vi "slider setter.vi"(6 "stepper motor state":T2, 7 "slider setter action":T3, 8 "state in":T1, 10 "value":dbl=1.0 format="%#_13g") -> (0 "state OUT":T1)   [LabVIEW 2018]
uses:
  slider setter action.ctl
  stepper motor state.ctl
  slider setter interal state.ctl
  2Dwindow.ctl
  stack action -- control.ctl
  slider action.ctl
  cursor action.ctl
  generate linear region.vi
  generate linear region --complex -- win cen.vi
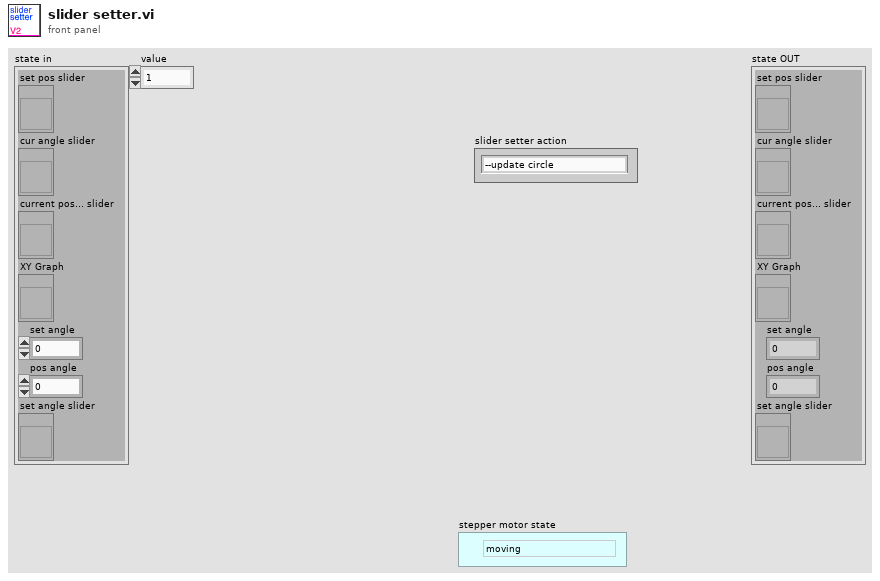
[diagram p1: front panel]
types:
  T1 = typedef "slider setter interal state.ctl" = cluster{"set pos slider":refnum<vi>, "cur angle slider":refnum<vi>, "current pos... slider":refnum<vi>, "XY Graph":refnum<vi>, "set angle":dbl, "pos angle":dbl, "set angle slider":refnum<vi>}
  T2 = typedef "stepper motor state.ctl" = enum16{"moving", "stopped"}
  T3 = typedef "slider setter action.ctl" = enum16{"--update circle", "set step slider moves", "cursor moves", "current pos changed", "init", "void", "--draw current lie", "--draw set line", "--move current step slider", "--move set step slider", "--draw limit lines", "check", "--move set angle slider", "--move current angle slider", "set angle slider moves", "--move cursor", "set set step", "set current step"}
  T4 = typedef "stack action -- control.ctl" = enum16{"push", "pop", "check", "init"}
  T5 = typedef "2Dwindow.ctl" = cluster{"window y":dbl, "center x":dbl, "center y":dbl, "window x":dbl}
  T6 = typedef "slider action.ctl" = enum16{"check", "copy range", "set from value", "set from ratio", "set from slider"}
  T7 = typedef "cursor action.ctl" = enum16{"range", "read", "write", "check", "zoom out", "smart zoom out", "zoom to aspect ratio 1", "zoom to win", "zoom out 20%", "zoom in 20%", "-empty", "smart zoom out&aspect", "move range left 20%", "move range right 20%", "move range up 20%", "move range down 20%", "zoom to X win", "zoom to Y win", "zoom out X", "zoom out Y", "zoom in X", "zoom in Y", "check plot scale"}
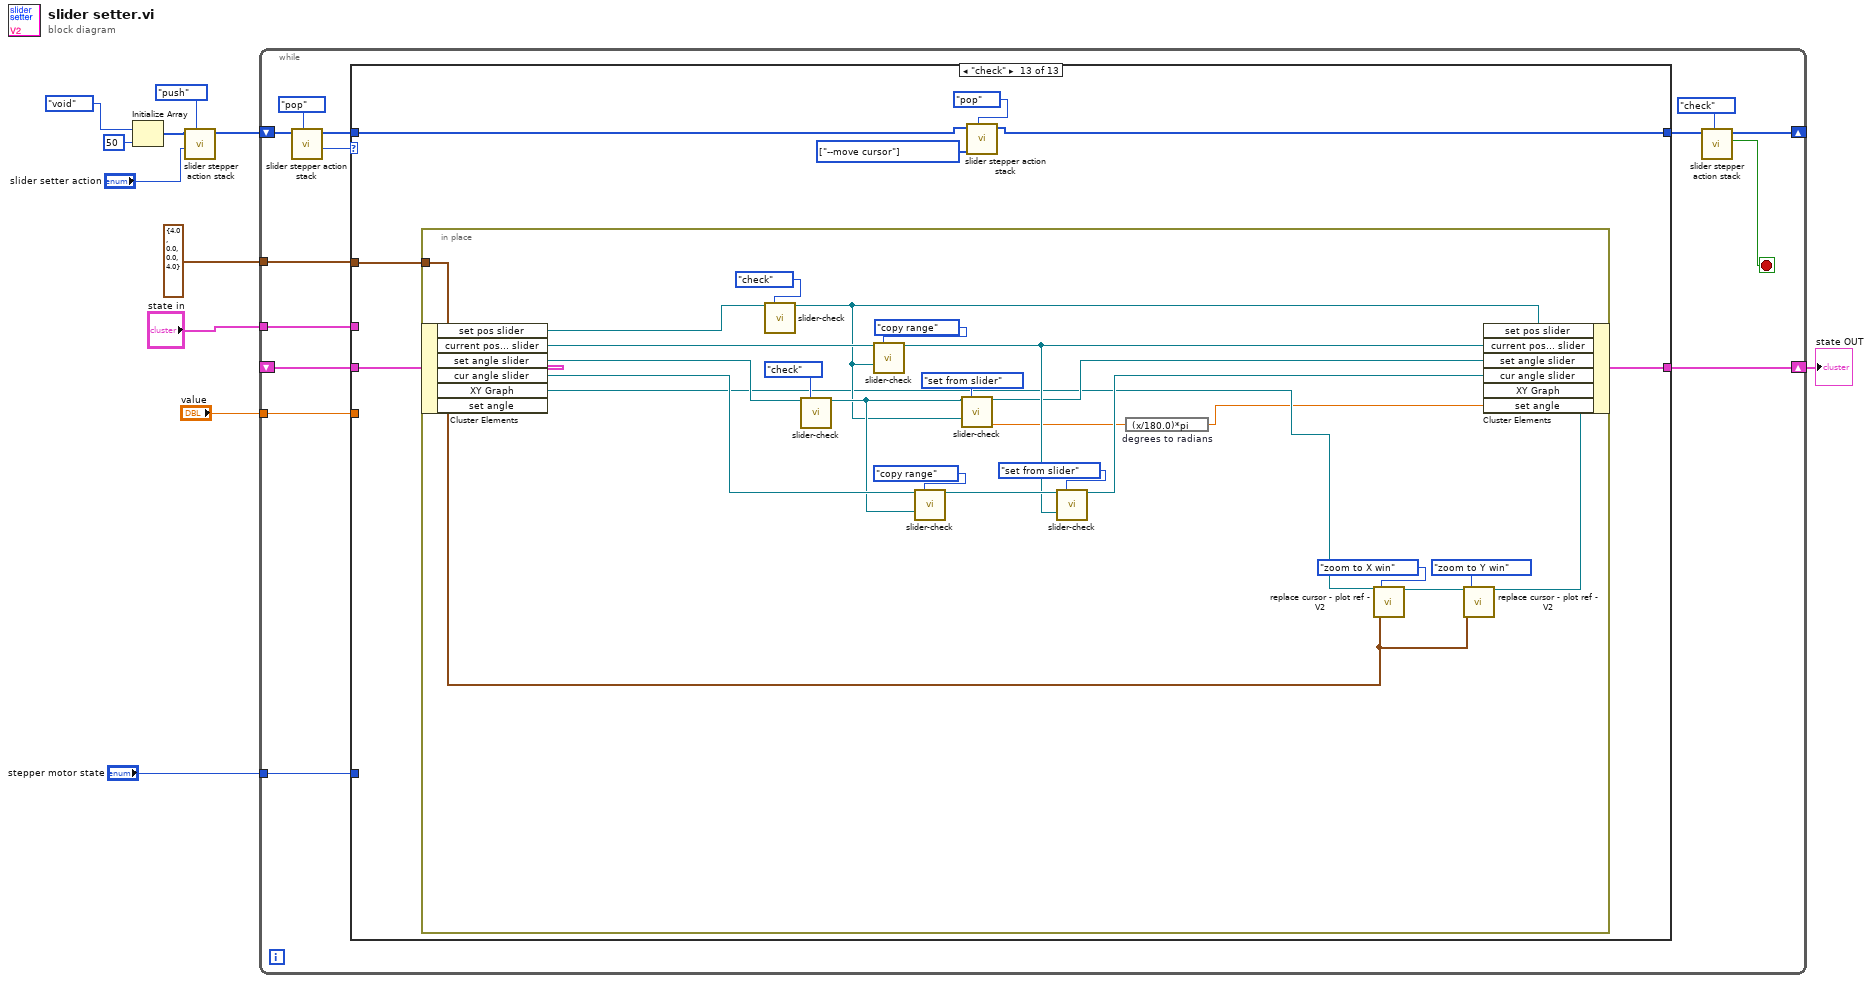
[diagram p0: block diagram]
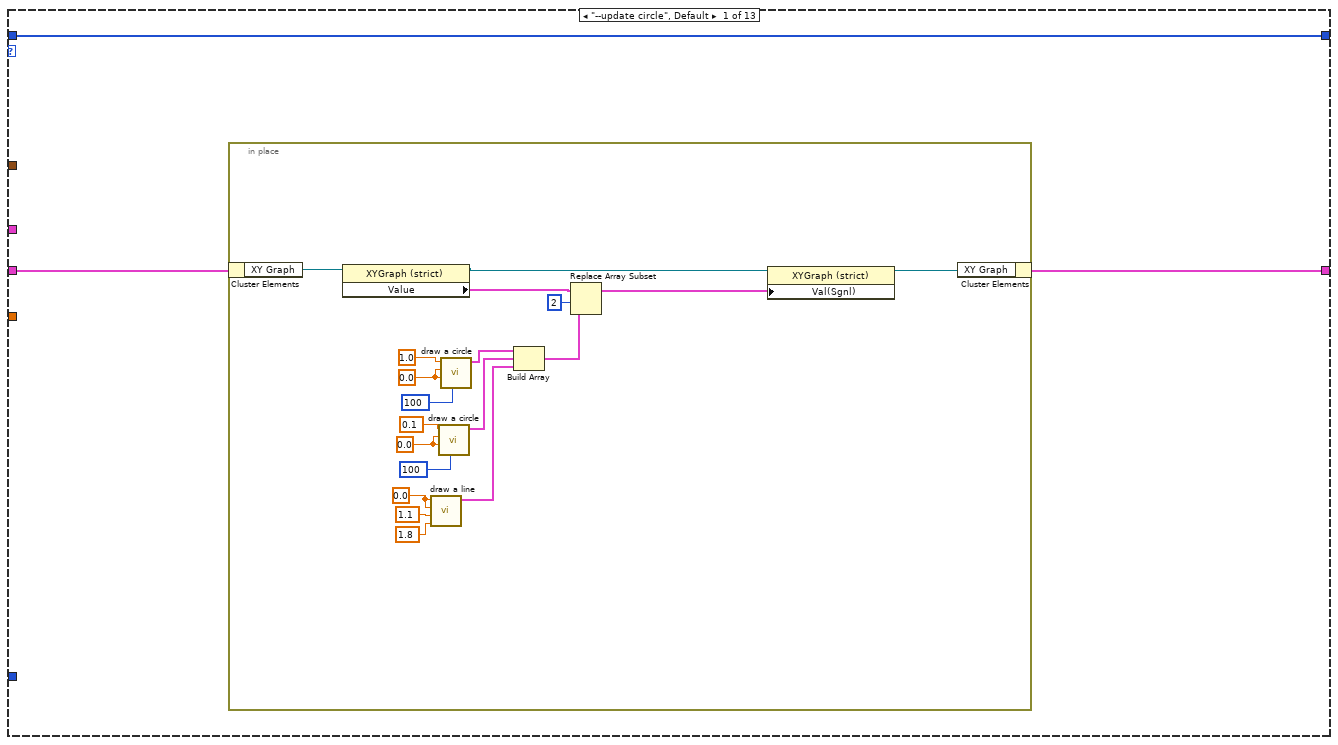
[diagram p2: hidden frame]
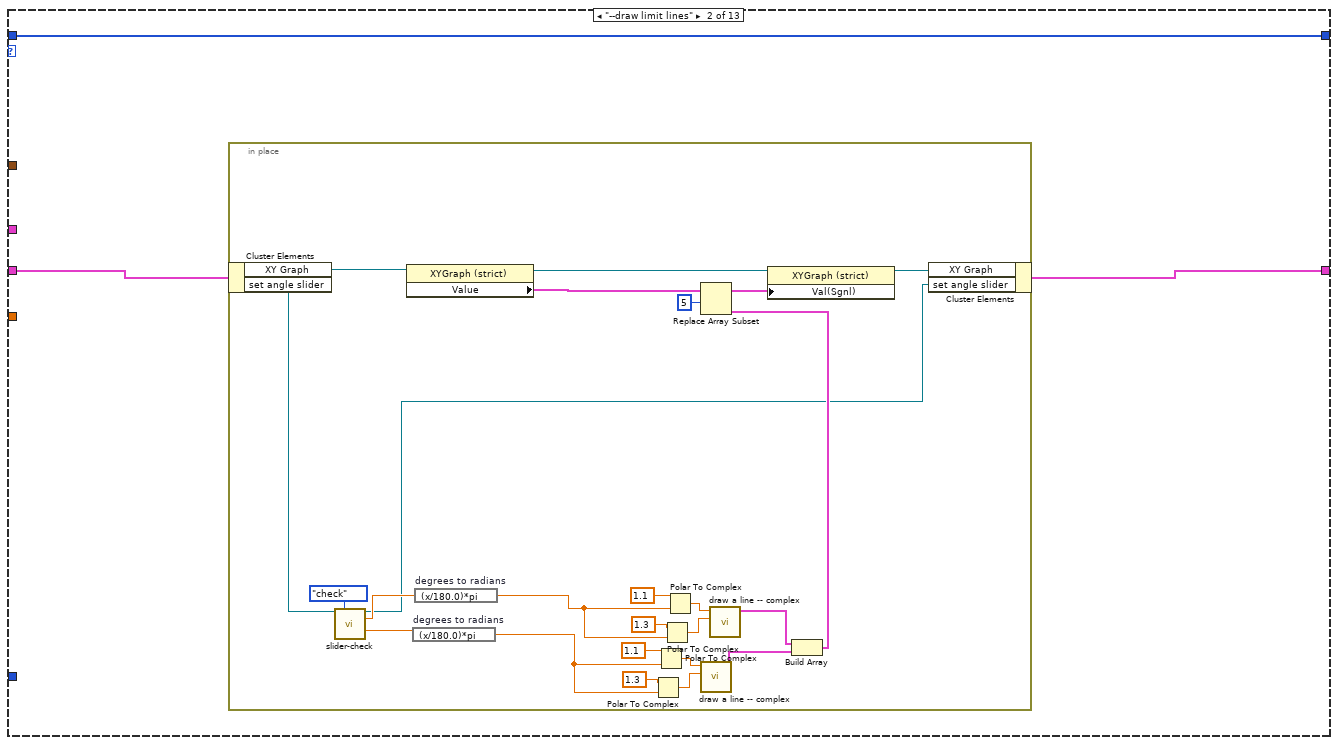
[diagram p3: hidden frame]
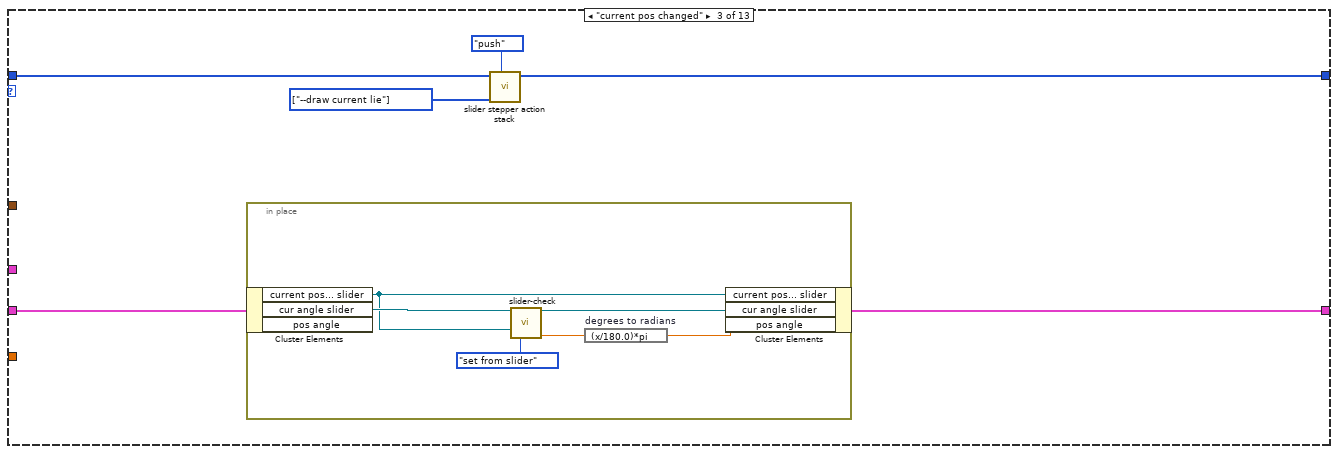
[diagram p4: hidden frame]
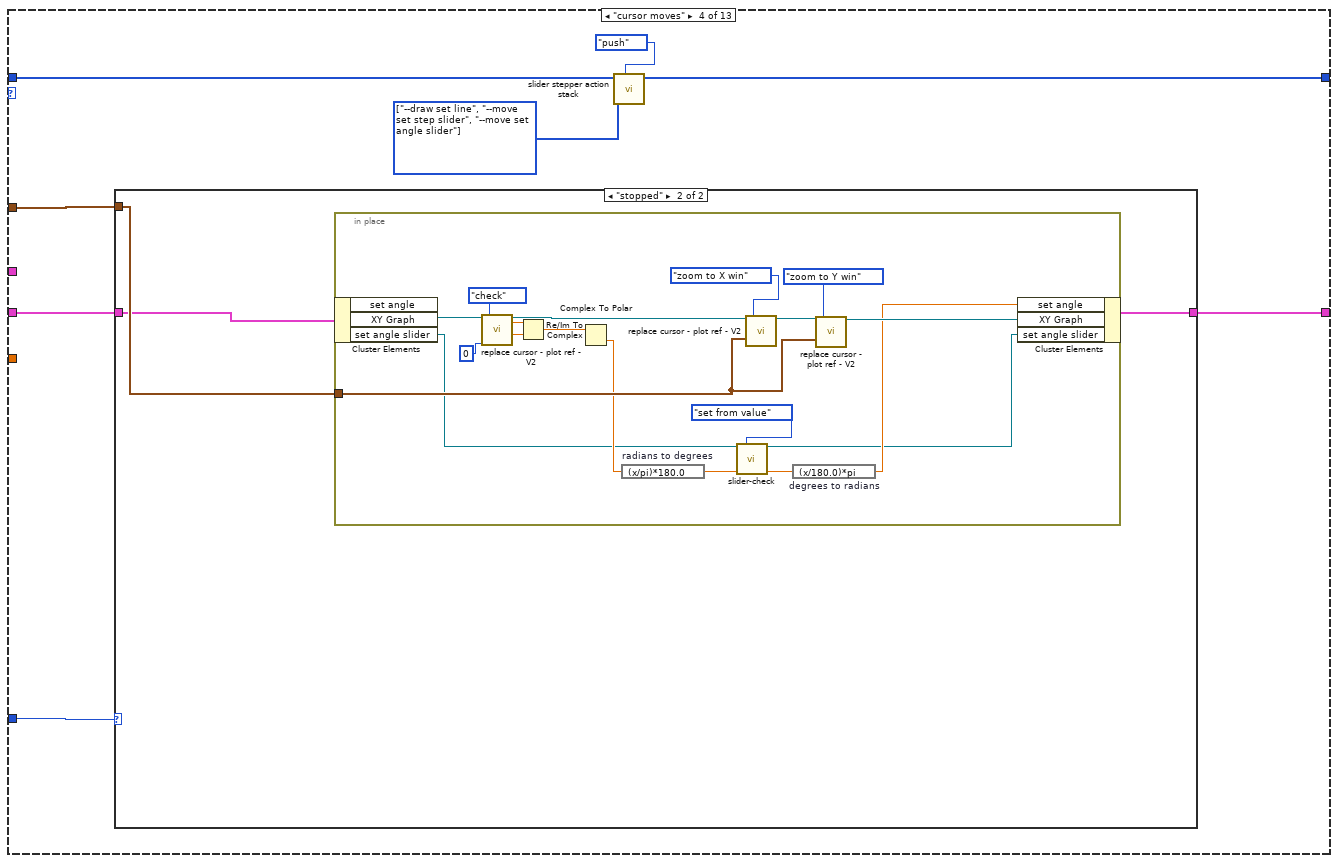
[diagram p5: hidden frame]
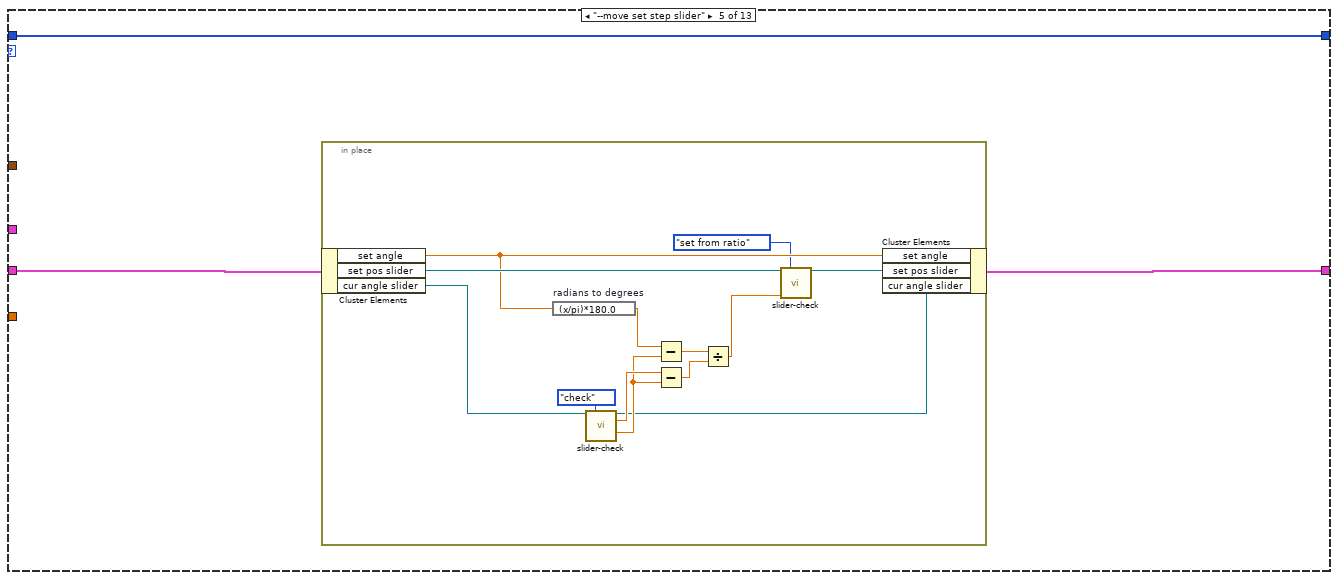
[diagram p7: hidden frame]
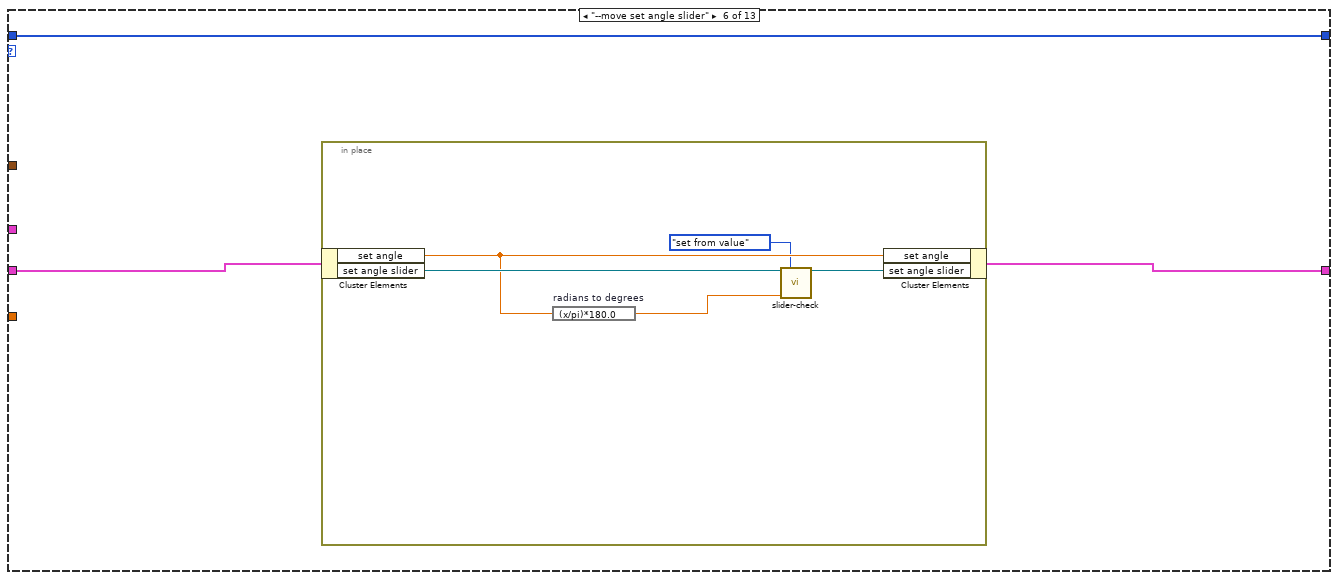
[diagram p8: hidden frame]
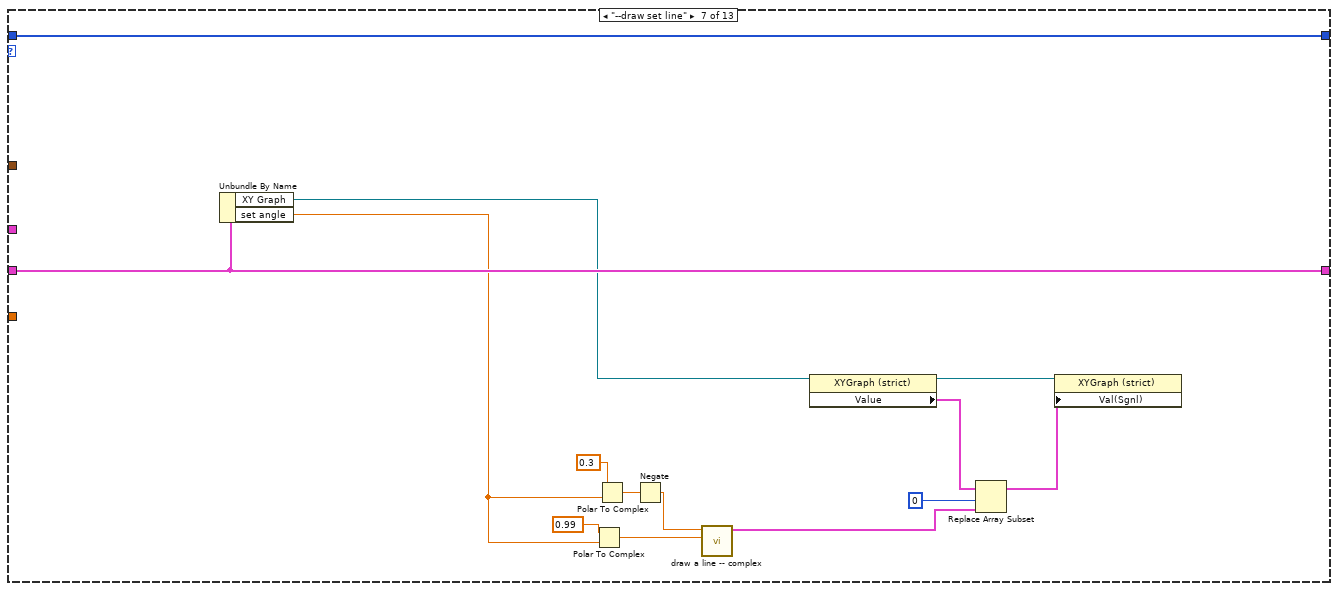
[diagram p9: hidden frame]
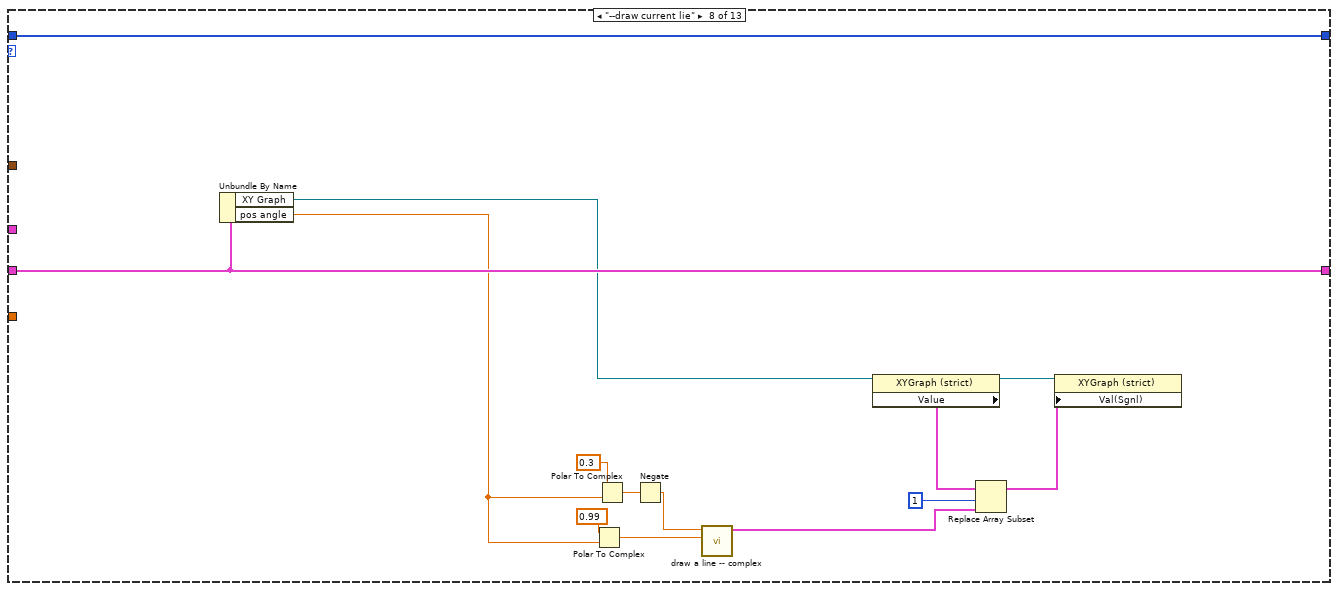
[diagram p10: hidden frame]
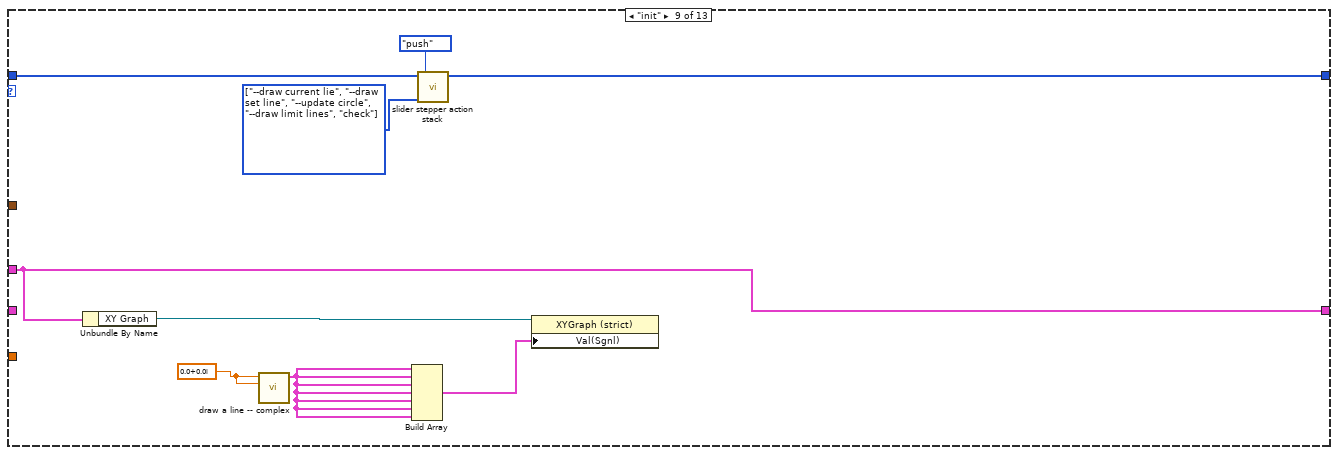
[diagram p11: hidden frame]
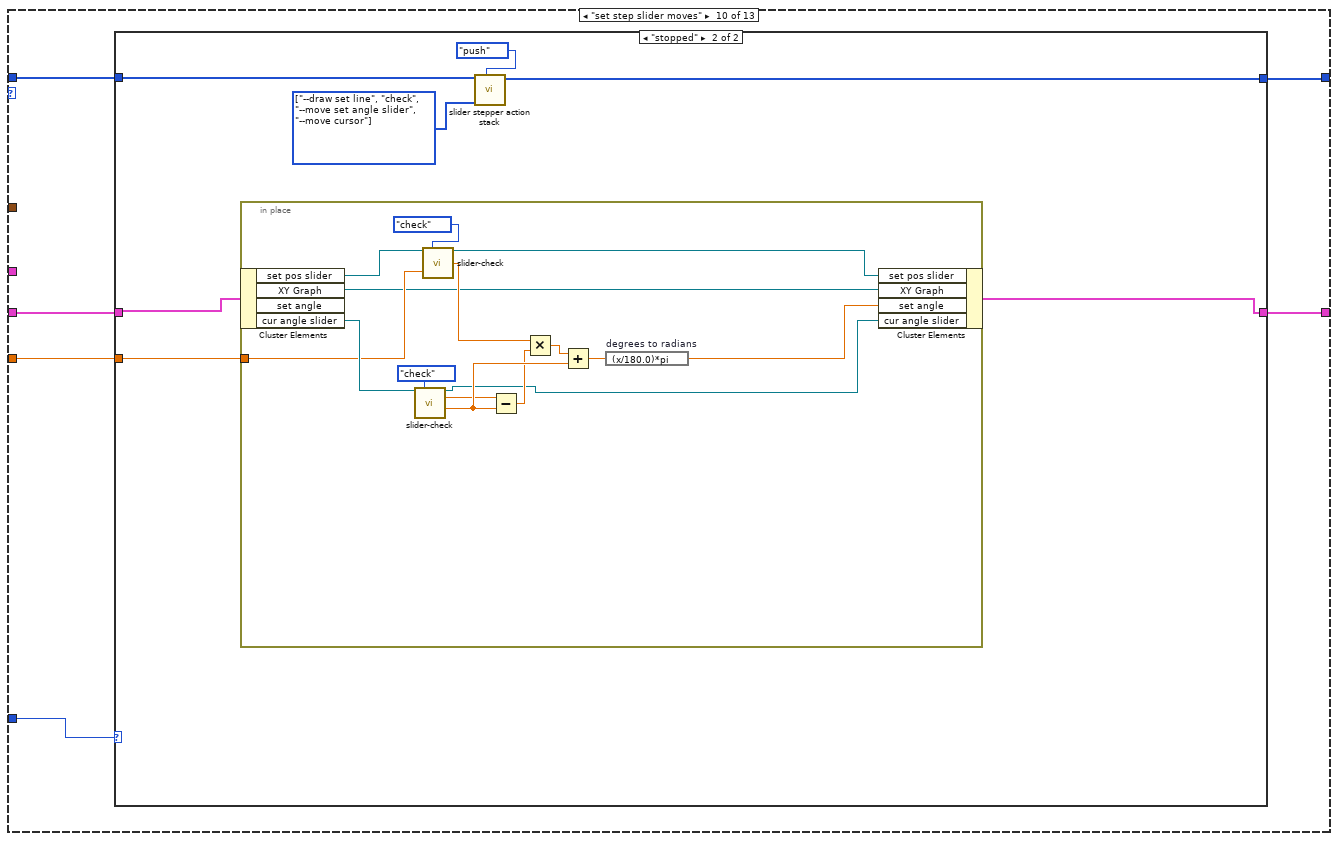
[diagram p12: hidden frame]
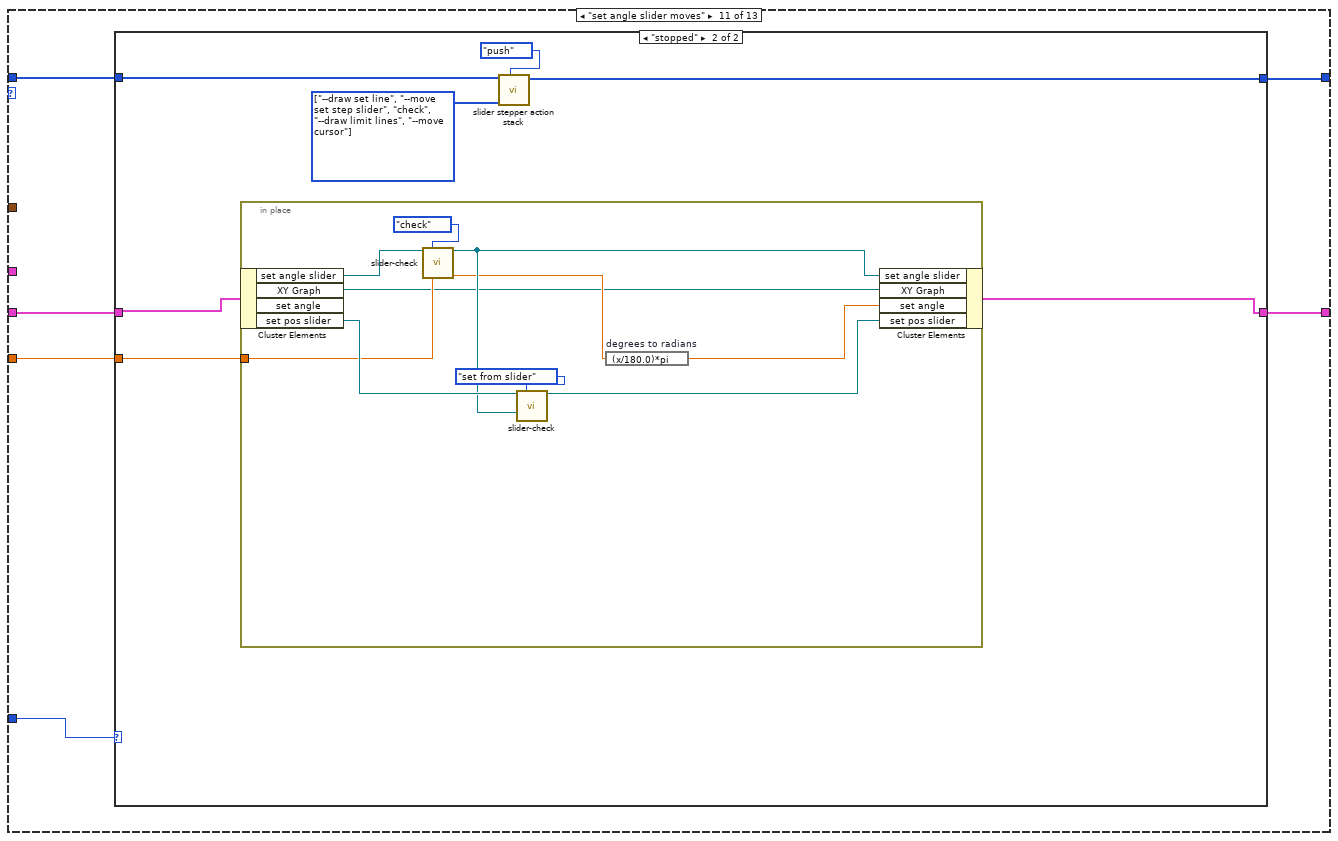
[diagram p14: hidden frame]
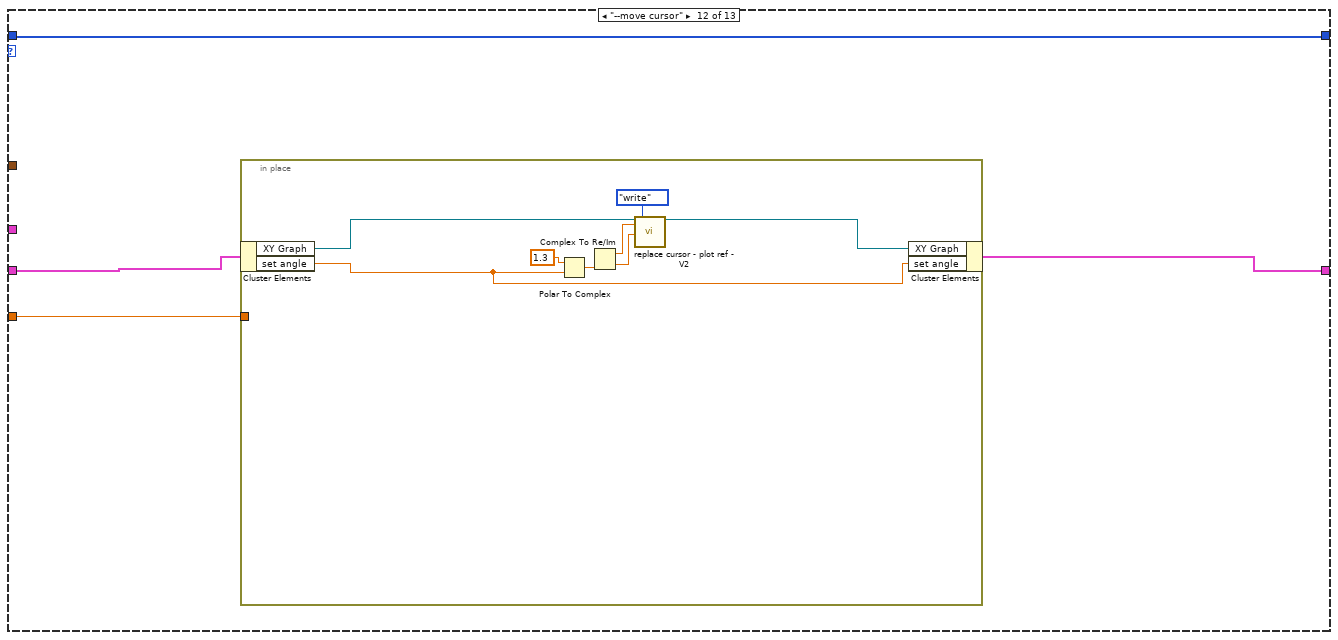
[diagram p16: hidden frame]
diagram:
  n1 = Initialize Array(slider_setter_action."void" ("slider setter action"), 50 ("dimension size")) -> (w7:T3[])
  n2 = call "slider stepper action stack.vi"("stack action"=stack_action_--_control."push", "slider setter action"="slider setter action", "command stack In"=w7) -> ("command stack OUT"=w5:T3[])  [unwired: 6 in, 2 out]
  n3 = while {
    tunnel: "stepper motor state" -> [w25]
    tunnel: T5 {"window y"=4.0, "center x"=0.0, "center y"=0.0, "window x"=4.0} ("window IN") -> [w24]
    shift-right: [w18] -> _
    shift-left: w5 -> [w22]
    tunnel: "state in" -> [w15]
    shift-right: [w14] -> w2
    shift-left: _ -> [w13]
    tunnel: "value" -> [w12]
    stop <- w16 stop-if-true
    n4 = call "slider stepper action stack.vi"("stack action"=stack_action_--_control."pop", "command stack In"=w22) -> ("slider setter action OUT"=w20:T3, "command stack OUT"=w21:T3[])  [unwired: 7 in, 1 out]
    n5 = case shown="\"check\"" w20 {
      tunnel: w25 -> [_ _ _ w94 _ _ _ _ _ w184 w214 _ _]
      tunnel: w24 -> [_ _ _ w93 _ _ _ _ _ _ _ _ w250]
      tunnel: w21 -> [w28 w50 w80 w91 w118 w134 w155 w169 w177 w183 w213 w234 w249]
      tunnel: [w28 w50 w79 w90 w118 w134 w155 w169 w176 w182 w212 w234 w248] -> w19
      tunnel: w15 -> [_ _ _ _ _ _ _ _ w171 _ _ _ _]
      tunnel: [w26 w48 w75 w89 w119 w135 w144 w158 w171 w181 w211 w237 w252] -> w14
      tunnel: w13 -> [w27 w49 w76 w88 w120 w136 w144 w158 _ w180 w210 w236 w251]
      tunnel: w12 -> [_ _ _ _ _ _ _ _ _ w179 w209 w235 _]
      frame "--update circle", Default {
        n6 = in-place {
          w41 = 0.0 ("center x")
          w44 = 0.0 ("x0")
          w47 = 0.0 ("center x")
          n7 = in-place-cluster #1(w27) -> ("XY Graph"=w37:refnum<vi>)
          n8 = property class="XYGraph (strict)"(reference=w37) -> (reference out=w36:refnum<vi>, "Value"=w35:cluster{dbl[], dbl[]}[])  [unwired: 1 in, 1 out]
          n9 = call "draw a line.vi"("y1"=1.8 ("x0"), "y0"=1.1 ("x0"), "x1"=w44, "x0"=w44) -> ("output cluster"=w31:cluster{dbl[], dbl[]})  [unwired: 7 in]
          n10 = call "draw a circle.vi"("number of points"=100, "center Y"=w41, "center x"=w41, "radius"=0.1) -> ("output cluster"=w32:cluster{dbl[], dbl[]})  [unwired: 7 in]
          n11 = call "draw a circle.vi"("number of points"=100, "center Y"=w47, "center x"=w47, "radius"=1.0) -> ("output cluster"=w33:cluster{dbl[], dbl[]})  [unwired: 7 in]
          n12 = Build Array(w33, w32, w31) -> (w30:cluster{dbl[], dbl[]}[])
          n13 = Replace Array Subset(array=w35, new element=w30, index=2) -> (w29:cluster{dbl[], dbl[]}[])
          n14 = property class="XYGraph (strict)"(reference=w36, "Val(Sgnl)"=w29) -> (reference out=w38:refnum<vi>)  [unwired: 1 in, 1 out]
          n15 = in-place-cluster #1("XY Graph"=w38) -> (w26:T1)
        }
      }
      frame "--draw limit lines" {
        n16 = in-place {
          n17 = in-place-cluster #2(w49) -> ("XY Graph"=w73:refnum<vi>, "set angle slider"=w67:refnum<vi>)
          n18 = call "slider-check.vi"("slider"=w67, "slider action"=slider_action."check") -> ("slider OUT"=w51:refnum<vi>, "max"=w66:dbl, "min"=w65:dbl)  [unwired: 9 in, 2 out]
          n19 = property class="XYGraph (strict)"(reference=w73) -> (reference out=w72:refnum<vi>, "Value"=w71:cluster{dbl[], dbl[]}[])  [unwired: 1 in, 1 out]
          n20 = expression code="(x/180.0)*pi" "degrees to radians"(w65) -> (w55:dbl)
          n21 = expression code="(x/180.0)*pi" "degrees to radians"(w66) -> (w61:dbl)
          n22 = Polar To Complex(1:w55, 2:1.3 ("x")) -> (0:w57:cdb)
          n23 = Polar To Complex(1:w55, 2:1.1 ("x")) -> (0:w56:cdb)
          n24 = Polar To Complex(1:w61, 2:1.3 ("x")) -> (0:w62:cdb)
          n25 = Polar To Complex(1:w61, 2:1.1 ("x")) -> (0:w60:cdb)
          n26 = call "draw a line -- complex.vi"("x1"=w57, "x0"=w56) -> ("output cluster"=w53:cluster{dbl[], dbl[]})  [unwired: 9 in]
          n27 = call "draw a line -- complex.vi"("x1"=w62, "x0"=w60) -> ("output cluster"=w54:cluster{dbl[], dbl[]})  [unwired: 9 in]
          n28 = Build Array(w54, w53) -> (w52:cluster{dbl[], dbl[]}[])
          n29 = Replace Array Subset(array=w71, new element=w52, index=5) -> (w69:cluster{dbl[], dbl[]}[])
          n30 = property class="XYGraph (strict)"(reference=w72, "Val(Sgnl)"=w69) -> (reference out=w74:refnum<vi>)  [unwired: 1 in, 1 out]
          n31 = in-place-cluster #2("XY Graph"=w74, "set angle slider"=w51) -> (w48:T1)
        }
      }
      frame "current pos changed" {
        w77 = T3[] [enum."--draw current lie"] items=["--update circle", "set step slider moves", "cursor moves", "current pos changed", "init", "void", "--draw current lie", "--draw set line", "--move current step slider", "--move set step slider", "--draw limit lines", "check", "--move set angle slider", "--move current angle slider", "set angle slider moves", "--move cursor", "set set step", "set current step"] ("action list IN")
        n32 = in-place {
          n33 = in-place-cluster #3(w76) -> ("current pos... slider"=w81:refnum<vi>, "cur angle slider"=w86:refnum<vi>)  [unwired: 1 out]
          n34 = call "slider-check.vi"("slider"=w86, "slider action"=slider_action."set from slider", "slider from"=w81) -> ("slider OUT"=w83:refnum<vi>, "value OUT"=w85:dbl)  [unwired: 8 in, 3 out]
          n35 = expression code="(x/180.0)*pi" "degrees to radians"(w85) -> (w84:dbl)
          n36 = in-place-cluster #3("current pos... slider"=w81, "cur angle slider"=w83, "pos angle"=w84) -> (w75:T1)
        }
        n37 = call "slider stepper action stack.vi"("stack action"=stack_action_--_control."push", "action list IN"=w77, "command stack In"=w80) -> ("command stack OUT"=w79:T3[])  [unwired: 6 in, 2 out]
      }
      frame "cursor moves" {
        w87 = T3[] [enum."--draw set line", enum."--move set step slider", enum."--move set angle slider"] items=["--update circle", "set step slider moves", "cursor moves", "current pos changed", "init", "void", "--draw current lie", "--draw set line", "--move current step slider", "--move set step slider", "--draw limit lines", "check", "--move set angle slider", "--move current angle slider", "set angle slider moves", "--move cursor", "set set step", "set current step"] ("action list IN")
        n38 = case shown="\"stopped\"" w94 {
          tunnel: w93 -> [_ w98]
          tunnel: [w95 w97] -> w89
          tunnel: w88 -> [w95 w96]
          frame "moving", Default {
          }
          frame "stopped" {
            n39 = in-place {
              in-place-border: w98 -> [w110]
              n40 = in-place-cluster #4(w96) -> ("XY Graph"=w108:refnum<vi>, "set angle slider"=w104:refnum<vi>)  [unwired: 1 out]
              n41 = call "replace cursor - plot ref - V2.vi"("Plot ref in"=w108, "cursor index"=0, "cursor action"=cursor_action."check") -> ("Plot ref out"=w109:refnum<vi>, "read X"=w115:dbl, "read Y"=w114:dbl)  [unwired: 13 in, 1 out]
              n42 = Re/Im To Complex(1:w114, 2:w115) -> (0:w113:cdb)
              n43 = Complex To Polar(r * e^(i*theta)=w113) -> (theta=w105:dbl)  [unwired: 1 out]
              n44 = expression code="(x/pi)*180.0" "radians to degrees"(w105) -> (w103:dbl)
              n45 = call "slider-check.vi"("slider"=w104, "slider action"=slider_action."set from value", "value IN"=w103) -> ("slider OUT"=w99:refnum<vi>, "value OUT"=w101:dbl)  [unwired: 8 in, 3 out]
              n46 = call "replace cursor - plot ref - V2.vi"("Plot ref in"=w109, "window IN"=w110, "cursor action"=cursor_action."zoom to X win") -> ("Plot ref out"=w107:refnum<vi>)  [unwired: 13 in, 3 out]
              n47 = expression code="(x/180.0)*pi" "degrees to radians"(w101) -> (w100:dbl)
              n48 = call "replace cursor - plot ref - V2.vi"("Plot ref in"=w107, "window IN"=w110, "cursor action"=cursor_action."zoom to Y win") -> ("Plot ref out"=w106:refnum<vi>)  [unwired: 13 in, 3 out]
              n49 = in-place-cluster #4("set angle"=w100, "XY Graph"=w106, "set angle slider"=w99) -> (w97:T1)
            }
          }
        }
        n50 = call "slider stepper action stack.vi"("stack action"=stack_action_--_control."push", "action list IN"=w87, "command stack In"=w91) -> ("command stack OUT"=w90:T3[])  [unwired: 6 in, 2 out]
      }
      frame "--move set step slider" {
        n51 = in-place {
          n52 = in-place-cluster #5(w120) -> ("set angle"=w123:dbl, "set pos slider"=w125:refnum<vi>, "cur angle slider"=w126:refnum<vi>)
          n53 = expression code="(x/pi)*180.0" "radians to degrees"(w123) -> (w127:dbl)
          n54 = call "slider-check.vi"("slider"=w126, "slider action"=slider_action."check") -> ("slider OUT"=w122:refnum<vi>, "max"=w132:dbl, "min"=w131:dbl)  [unwired: 9 in, 2 out]
          n55 = Subtract(x=w127, y=w131) -> (x-y=w130:dbl)
          n56 = Subtract(x=w132, y=w131) -> (x-y=w129:dbl)
          n57 = Divide(x=w130, y=w129) -> (x/y=w128:dbl)
          n58 = call "slider-check.vi"("slider"=w125, "slider action"=slider_action."set from ratio", "value IN"=w128) -> ("slider OUT"=w124:refnum<vi>)  [unwired: 8 in, 4 out]
          n59 = in-place-cluster #5("set angle"=w123, "set pos slider"=w124, "cur angle slider"=w122) -> (w119:T1)
        }
      }
      frame "--move set angle slider" {
        n60 = in-place {
          n61 = in-place-cluster #6(w136) -> ("set angle"=w139:dbl, "set angle slider"=w141:refnum<vi>)
          n62 = expression code="(x/pi)*180.0" "radians to degrees"(w139) -> (w138:dbl)
          n63 = call "slider-check.vi"("slider"=w141, "slider action"=slider_action."set from value", "value IN"=w138) -> ("slider OUT"=w140:refnum<vi>)  [unwired: 8 in, 4 out]
          n64 = in-place-cluster #6("set angle"=w139, "set angle slider"=w140) -> (w135:T1)
        }
      }
      frame "--draw set line" {
        n65 = Unbundle By Name(w144) -> ("XY Graph"=w142:refnum<vi>, "set angle"=w143:dbl)
        n66 = Polar To Complex(1:w143, 2:0.99 ("x")) -> (0:w146:cdb)
        n67 = Polar To Complex(1:w143, 2:0.3 ("x")) -> (0:w148:cdb)
        n68 = Negate(x=w148) -> (-x=w147:cdb)
        n69 = call "draw a line -- complex.vi"("x1"=w146, "x0"=w147) -> ("output cluster"=w145:cluster{dbl[], dbl[]})  [unwired: 9 in]
        n70 = property class="XYGraph (strict)"(reference=w142) -> (reference out=w154:refnum<vi>, "Value"=w153:cluster{dbl[], dbl[]}[])  [unwired: 1 in, 1 out]
        n71 = Replace Array Subset(array=w153, new element=w145, index=0) -> (w152:cluster{dbl[], dbl[]}[])
        n72 = property class="XYGraph (strict)"(reference=w154, "Val(Sgnl)"=w152) -> ()  [unwired: 1 in, 2 out]
      }
      frame "--draw current lie" {
        n73 = Unbundle By Name(w158) -> ("XY Graph"=w156:refnum<vi>, "pos angle"=w157:dbl)
        n74 = Polar To Complex(1:w157, 2:0.99 ("x")) -> (0:w160:cdb)
        n75 = Polar To Complex(1:w157, 2:0.3 ("x")) -> (0:w162:cdb)
        n76 = Negate(x=w162) -> (-x=w161:cdb)
        n77 = call "draw a line -- complex.vi"("x1"=w160, "x0"=w161) -> ("output cluster"=w159:cluster{dbl[], dbl[]})  [unwired: 9 in]
        n78 = property class="XYGraph (strict)"(reference=w156) -> (reference out=w168:refnum<vi>, "Value"=w167:cluster{dbl[], dbl[]}[])  [unwired: 1 in, 1 out]
        n79 = Replace Array Subset(array=w167, new element=w159, index=1) -> (w166:cluster{dbl[], dbl[]}[])
        n80 = property class="XYGraph (strict)"(reference=w168, "Val(Sgnl)"=w166) -> ()  [unwired: 1 in, 2 out]
      }
      frame "init" {
        w173 = cdb 0.0+0.0i ("x0")
        w174 = T3[] [enum."--draw current lie", enum."--draw set line", enum."--update circle", enum."--draw limit lines", enum."check"] items=["--update circle", "set step slider moves", "cursor moves", "current pos changed", "init", "void", "--draw current lie", "--draw set line", "--move current step slider", "--move set step slider", "--draw limit lines", "check", "--move set angle slider", "--move current angle slider", "set angle slider moves", "--move cursor", "set set step", "set current step"] ("action list IN")
        n81 = Unbundle By Name(w171) -> ("XY Graph"=w170:refnum<vi>)
        n82 = call "draw a line -- complex.vi"("x1"=w173, "x0"=w173) -> ("output cluster"=w172:cluster{dbl[], dbl[]})  [unwired: 9 in]
        n83 = Build Array(w172, w172, w172, w172, w172, w172, w172) -> (w178:cluster{dbl[], dbl[]}[])
        n84 = call "slider stepper action stack.vi"("stack action"=stack_action_--_control."push", "action list IN"=w174, "command stack In"=w177) -> ("command stack OUT"=w176:T3[])  [unwired: 6 in, 2 out]
        n85 = property class="XYGraph (strict)"(reference=w170, "Val(Sgnl)"=w178) -> ()  [unwired: 1 in, 2 out]
      }
      frame "set step slider moves" {
        n86 = case shown="\"stopped\"" w184 {
          tunnel: w183 -> [w186 w193]
          tunnel: [w186 w192] -> w182
          tunnel: w180 -> [w185 w190]
          tunnel: [w185 w189] -> w181
          tunnel: w179 -> [_ w187]
          frame "moving", Default {
          }
          frame "stopped" {
            w191 = T3[] [enum."--draw set line", enum."check", enum."--move set angle slider", enum."--move cursor"] items=["--update circle", "set step slider moves", "cursor moves", "current pos changed", "init", "void", "--draw current lie", "--draw set line", "--move current step slider", "--move set step slider", "--draw limit lines", "check", "--move set angle slider", "--move current angle slider", "set angle slider moves", "--move cursor", "set set step", "set current step"] ("action list IN")
            n87 = in-place {
              in-place-border: w187 -> [w196]
              n88 = in-place-cluster #7(w190) -> ("set pos slider"=w202:refnum<vi>, "XY Graph"=w194:refnum<vi>, "cur angle slider"=w201:refnum<vi>)  [unwired: 1 out]
              n89 = call "slider-check.vi"("slider"=w201, "slider action"=slider_action."check") -> ("slider OUT"=w197:refnum<vi>, "max"=w205:dbl, "min"=w208:dbl)  [unwired: 9 in, 2 out]
              n90 = call "slider-check.vi"("slider"=w202, "slider action"=slider_action."check", "default"=w196) -> ("slider OUT"=w198:refnum<vi>, "rel OUT"=w199:dbl)  [unwired: 8 in, 3 out]
              n91 = Subtract(x=w205, y=w208) -> (x-y=w206:dbl)
              n92 = Multiply(x=w199, y=w206) -> (x*y=w207:dbl)
              n93 = Add(x=w207, y=w208) -> (x+y=w195:dbl)
              n94 = expression code="(x/180.0)*pi" "degrees to radians"(w195) -> (w200:dbl)
              n95 = in-place-cluster #7("set pos slider"=w198, "XY Graph"=w194, "set angle"=w200, "cur angle slider"=w197) -> (w189:T1)
            }
            n96 = call "slider stepper action stack.vi"("stack action"=stack_action_--_control."push", "action list IN"=w191, "command stack In"=w193) -> ("command stack OUT"=w192:T3[])  [unwired: 6 in, 2 out]
          }
        }
      }
      frame "set angle slider moves" {
        n97 = case shown="\"stopped\"" w214 {
          tunnel: w213 -> [w216 w223]
          tunnel: [w216 w222] -> w212
          tunnel: w210 -> [w215 w220]
          tunnel: [w215 w219] -> w211
          tunnel: w209 -> [_ w217]
          frame "moving", Default {
          }
          frame "stopped" {
            w221 = T3[] [enum."--draw set line", enum."--move set step slider", enum."check", enum."--draw limit lines", enum."--move cursor"] items=["--update circle", "set step slider moves", "cursor moves", "current pos changed", "init", "void", "--draw current lie", "--draw set line", "--move current step slider", "--move set step slider", "--draw limit lines", "check", "--move set angle slider", "--move current angle slider", "set angle slider moves", "--move cursor", "set set step", "set current step"] ("action list IN")
            n98 = in-place {
              in-place-border: w217 -> [w228]
              n99 = in-place-cluster #8(w220) -> ("set angle slider"=w231:refnum<vi>, "XY Graph"=w224:refnum<vi>, "set pos slider"=w230:refnum<vi>)  [unwired: 1 out]
              n100 = call "slider-check.vi"("slider"=w231, "slider action"=slider_action."check", "default"=w228) -> ("slider OUT"=w227:refnum<vi>, "value OUT"=w225:dbl)  [unwired: 8 in, 3 out]
              n101 = call "slider-check.vi"("slider"=w230, "slider action"=slider_action."set from slider", "slider from"=w227) -> ("slider OUT"=w226:refnum<vi>)  [unwired: 8 in, 4 out]
              n102 = expression code="(x/180.0)*pi" "degrees to radians"(w225) -> (w229:dbl)
              n103 = in-place-cluster #8("set angle slider"=w227, "XY Graph"=w224, "set angle"=w229, "set pos slider"=w226) -> (w219:T1)
            }
            n104 = call "slider stepper action stack.vi"("stack action"=stack_action_--_control."push", "action list IN"=w221, "command stack In"=w223) -> ("command stack OUT"=w222:T3[])  [unwired: 6 in, 2 out]
          }
        }
      }
      frame "--move cursor" {
        n105 = in-place {
          in-place-border: w235 -> [_]
          n106 = in-place-cluster #9(w236) -> ("XY Graph"=w240:refnum<vi>, "set angle"=w238:dbl)
          n107 = Polar To Complex(1:w238, 2:1.3 ("r")) -> (0:w243:cdb)
          n108 = Complex To Re/Im(x + iy=w243) -> (x=w244:dbl, y=w245:dbl)
          n109 = call "replace cursor - plot ref - V2.vi"("Plot ref in"=w240, "new X"=w244, "new  Y"=w245, "cursor action"=cursor_action."write") -> ("Plot ref out"=w239:refnum<vi>)  [unwired: 12 in, 3 out]
          n110 = in-place-cluster #9("XY Graph"=w239, "set angle"=w238) -> (w237:T1)
        }
      }
      frame "check" {
        w246 = T3[] [enum."--move cursor"] items=["--update circle", "set step slider moves", "cursor moves", "current pos changed", "init", "void", "--draw current lie", "--draw set line", "--move current step slider", "--move set step slider", "--draw limit lines", "check", "--move set angle slider", "--move current angle slider", "set angle slider moves", "--move cursor", "set set step", "set current step"] ("action list IN")
        n111 = in-place {
          in-place-border: w250 -> [w257]
          n112 = in-place-cluster #10(w251) -> ("set pos slider"=w274:refnum<vi>, "current pos... slider"=w272:refnum<vi>, "set angle slider"=w271:refnum<vi>, "cur angle slider"=w270:refnum<vi>, "XY Graph"=w254:refnum<vi>)  [unwired: 1 out]
          n113 = call "slider-check.vi"("slider"=w274, "slider action"=slider_action."check") -> ("slider OUT"=w261:refnum<vi>)  [unwired: 9 in, 4 out]
          n114 = call "slider-check.vi"("slider"=w271, "slider action"=slider_action."check") -> ("slider OUT"=w263:refnum<vi>)  [unwired: 9 in, 4 out]
          n115 = call "slider-check.vi"("slider"=w272, "slider action"=slider_action."copy range", "slider from"=w261) -> ("slider OUT"=w265:refnum<vi>)  [unwired: 8 in, 4 out]
          n116 = call "slider-check.vi"("slider"=w270, "slider action"=slider_action."copy range", "slider from"=w263) -> ("slider OUT"=w268:refnum<vi>)  [unwired: 8 in, 4 out]
          n117 = call "slider-check.vi"("slider"=w263, "slider action"=slider_action."set from slider", "slider from"=w261) -> ("slider OUT"=w262:refnum<vi>, "value OUT"=w258:dbl)  [unwired: 8 in, 3 out]
          n118 = call "slider-check.vi"("slider"=w268, "slider action"=slider_action."set from slider", "slider from"=w265) -> ("slider OUT"=w267:refnum<vi>)  [unwired: 8 in, 4 out]
          n119 = expression code="(x/180.0)*pi" "degrees to radians"(w258) -> (w253:dbl)
          n120 = call "replace cursor - plot ref - V2.vi"("Plot ref in"=w254, "window IN"=w257, "cursor action"=cursor_action."zoom to X win") -> ("Plot ref out"=w259:refnum<vi>)  [unwired: 13 in, 3 out]
          n121 = call "replace cursor - plot ref - V2.vi"("Plot ref in"=w259, "window IN"=w257, "cursor action"=cursor_action."zoom to Y win") -> ("Plot ref out"=w256:refnum<vi>)  [unwired: 13 in, 3 out]
          n122 = in-place-cluster #10("set pos slider"=w261, "current pos... slider"=w265, "set angle slider"=w262, "cur angle slider"=w267, "XY Graph"=w256, "set angle"=w253) -> (w252:T1)
        }
        n123 = call "slider stepper action stack.vi"("stack action"=stack_action_--_control."pop", "action list IN"=w246, "command stack In"=w249) -> ("command stack OUT"=w248:T3[])  [unwired: 6 in, 2 out]
      }
    }
    n124 = call "slider stepper action stack.vi"("stack action"=stack_action_--_control."check", "command stack In"=w19) -> ("stack is empty ?"=w16:bool, "command stack OUT"=w18:T3[])  [unwired: 7 in, 1 out]
  }
  "state OUT" <- w2
